vi "q3 plots.vi"() -> ()   [LabVIEW 2018]
uses:
  <vilib>/addons/Control Design/_Utility/Rendering.llb/Rendering Transfer Function Options.ctl
  <vilib>/addons/Control Design/_Model Construction/Data Typedefs.llb/CD Bode Data.ctl
  <vilib>/addons/Control Design/_Model Construction/Data Typedefs.llb/CD Plot Types Enum.ctl
  <vilib>/addons/Control Design/_Model Construction/Data Typedefs.llb/CD Root Locus with Gain Info.ctl
  <vilib>/addons/Control Design/_Model Construction/Model Creation.llb/Model Creation SubVI/cd_Create Transfer Function Model.vi
  <vilib>/addons/Control Design/_Model Conversions/Model Type.llb/Model Conversion SubVI/cd_Convert Transfer Function to State-Space Model.vi
  <vilib>/addons/Control Design/_Dynamic Analysis/Dynamic Analysis.llb/Dynamic Analysis subVI/cd_Root Locus (State-Space).vi
  <vilib>/addons/Control Design/_Dynamic Analysis/Dynamic Analysis.llb/Dynamic Analysis subVI/cd_Stability (State-Space).vi
  <vilib>/addons/Control Design/_Frequency Response Analysis/Frequency Response.llb/Frequency Response subVI/cd_Bode (State Space).vi
  <vilib>/addons/Control Design/_Utility/Model Viewer.llb/Model Viewer SubVI/cd_Draw State-Space Equation (SS).vi
  <vilib>/addons/Control Design/_Utility/Model Viewer.llb/Model Viewer SubVI/cd_Draw Transfer Function Equation (TF).vi
  <vilib>/addons/Control Design/_Model Construction/NI_LinSys_Model Creation.lvlib
  <vilib>/addons/Control Design/_Utility/NI_CD_Model Viewer.lvlib
  <vilib>/addons/Control Design/_Model Conversions/NI_CD_Model Type.lvlib
  <vilib>/addons/Control Design/_Frequency Response Analysis/NI_CD_Frequency Response.lvlib
  <vilib>/addons/Control Design/_Dynamic Analysis/NI_CD_Dynamic Analysis.lvlib
  <vilib>/addons/Control Design/_Utility/NI_LinSys_Rendering.lvlib
  <vilib>/addons/Control Design/_Model Construction/NI_LinSys_Data Typedefs.lvlib
panel:
  out "Root Locus Information":T1
  out "Root Locus Data":cluster{"K":dbl[], "Roots":cdb[][]} {"Roots" format="%.2f"; "K" format="%.4f"}
  out "Root Locus Graph":cluster{dbl[], dbl[]}[](graph)
  out "Poles":cdb[](array[numeric]) format="%.2e"
  out "Stability":T2(ring)=enum."undetermined"
  out "Bode Data":T3={"Frequency"=[], "Magnitude"=[], "Phase"=[], "plot type"=enum."bode-phase"} {"Phase" format="%#.6g"; "Magnitude" format="%#.6g"; "Frequency" format="%#.6g"}
  out "Bode Phase":cluster{"W":dbl[], "Magnitude":dbl[]}[](graph)
  out "Bode Magnitude":cluster{"W":dbl[], "Magnitude":dbl[]}[](graph)
  out "State Space":picture
  out "Transfer Function":picture
  in  "Display Format":T5 items=["Descending", "Ascending", "Negative Power"]
  in  "Denominator":dbl[](array[numeric]) format="%#.5g"
  in  "Numerator":dbl[](array[numeric]) format="%#.5g"
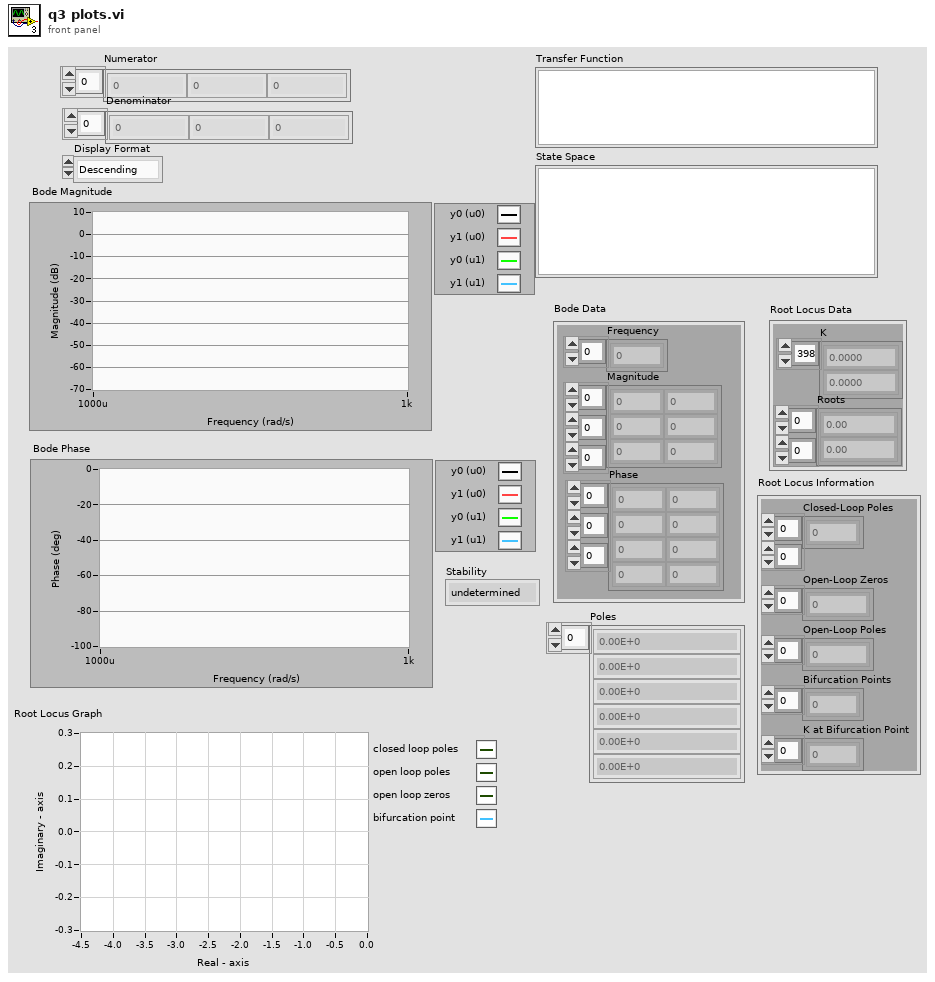
[diagram p1: front panel]
types:
  T1 = typedef "NI_LinSys_Data Typedefs.lvlib/CD Root Locus with Gain Info.ctl" = cluster{"Closed-Loop Poles":cdb[][], "Open-Loop Zeros":cdb[], "Open-Loop Poles":cdb[], "Bifurcation Points":cdb[], "K at Bifurcation Point":dbl[]}
  T2 = enum16{"stable", "marginally stable", "unstable", "undetermined"}
  T3 = typedef "NI_LinSys_Data Typedefs.lvlib/CD Bode Data.ctl" = cluster{"Frequency":dbl[], "Magnitude":dbl[][][], "Phase":dbl[][][], "plot type":T4}
  T4 = typedef "NI_LinSys_Data Typedefs.lvlib/CD Plot Types Enum.ctl" = enum16{"bode-magnitude", "bode-phase", "nichols", "nyquist", "singular values", "step", "impulse", "initial", "simulation", "nyquist with separation"}
  T5 = typedef "NI_LinSys_Rendering.lvlib/Rendering Transfer Function Options.ctl" = u16
  T6 = typedef "NI_LinSys_Model Typedefs.lvlib/CD Transfer Function Model (MIMO).ctl" = cluster{"properties":T7, "transfer function(s)":T8[][]}
  T7 = typedef "NI_LinSys_Model Typedefs.lvlib/CD General Elements.ctl" = cluster{"Model name":string, "Input names":string[], "Output names":string[], "Input Delays":dbl[], "Output Delays":dbl[], "Sampling Time":dbl, "Notes":string}
  T8 = typedef "NI_LinSys_Model Typedefs.lvlib/CD Transfer Function Model (SISO).ctl" = cluster{"Numerator":dbl[], "Denominator":dbl[], "delay":dbl}
  T9 = typedef "NI_LinSys_Model Typedefs.lvlib/CD State Space Model (MIMO).ctl" = cluster{"properties":T7, "A":dbl[][], "B":dbl[][], "C":dbl[][], "D":dbl[][], "StateNames":string[], "Transport Delay":dbl[][]}
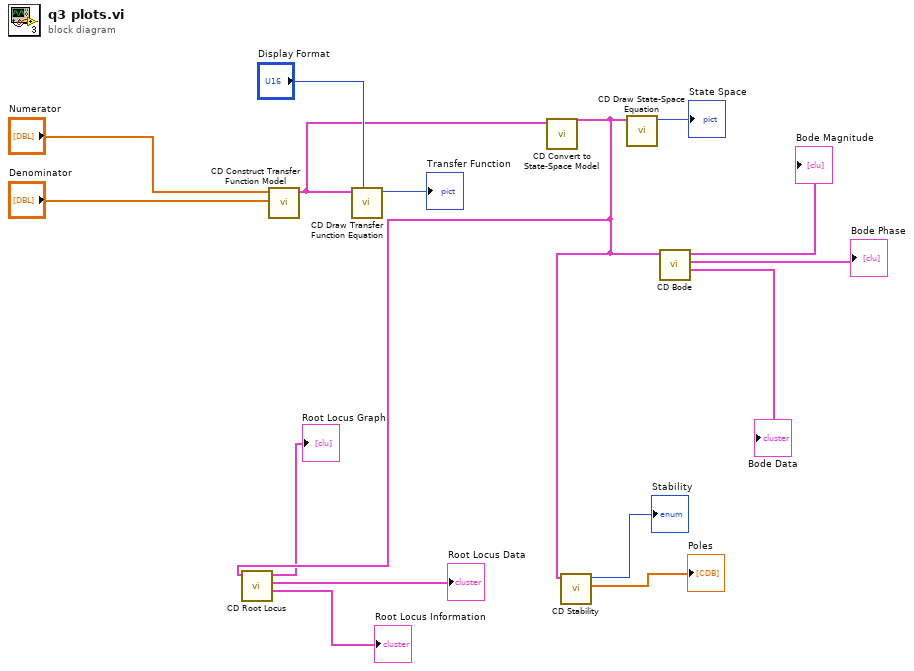
[diagram p0: block diagram]
diagram:
  n1 = call-poly <vilib>:"CD Construct Transfer Function Model.vi"("Denominator"="Denominator", "Numerator"="Numerator") -> ("Transfer Function Model"=w11:T6)  [unwired: 8 in, 1 out]
  n2 = call-poly <vilib>:"CD Draw Transfer Function Equation.vi"("Display Format"="Display Format", "Transfer Function Model"=w11) -> ("Equation"=→"Transfer Function":picture)  [unwired: 7 in, 2 out]
  n3 = call-poly <vilib>:"CD Convert to State-Space Model.vi"("Transfer Function Model"=w11) -> ("State-Space Model"=w4:T9)  [unwired: 9 in, 1 out]
  n4 = call-poly <vilib>:"CD Root Locus.vi"("State-Space Model"=w4) -> ("Root Locus Information"=→"Root Locus Information":T1, "Root Locus Data"=→"Root Locus Data":cluster{"K":dbl[], "Roots":cdb[][]}, "Root Locus Graph"=→"Root Locus Graph":cluster{dbl[], dbl[]}[])  [unwired: 7 in, 1 out]
  n5 = call-poly <vilib>:"CD Stability.vi"("State-Space Model"=w4) -> ("Poles"=→"Poles":cdb[], "Stability"=→"Stability":T2)  [unwired: 8 in, 1 out]
  n6 = call-poly <vilib>:"CD Draw State-Space Equation.vi"("State-Space Model"=w4) -> ("Equation"=→"State Space":picture)  [unwired: 8 in, 2 out]
  n7 = call-poly <vilib>:"CD Bode.vi"("State-Space Model"=w4) -> ("Bode Data"=→"Bode Data":T3, "Bode Phase"=→"Bode Phase":cluster{"W":dbl[], "Magnitude":dbl[]}[], "Bode Magnitude"=→"Bode Magnitude":cluster{"W":dbl[], "Magnitude":dbl[]}[])  [unwired: 6 in, 2 out]
